vi "Initialise Singleton.vi"(8 "error in (no error)":errorcluster, 11 "Class in":refnum<class>) -> (0 "error out":errorcluster)   [LabVIEW 2020, in "Singleton.lvlib"]
uses:
  Singleton.lvlib
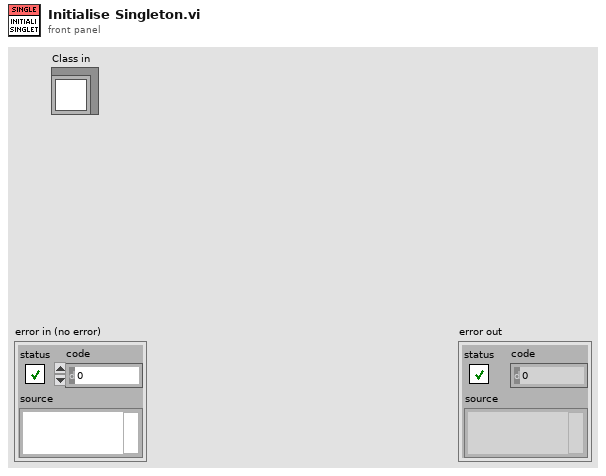
[diagram p1: front panel]
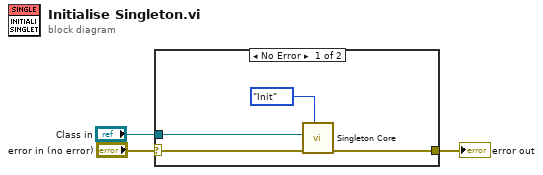
[diagram p0: block diagram]
diagram:
  n1 = case shown="No Error" "error in (no error)" {
    selector: "error in (no error)" -> [w7 w8]
    tunnel: [w6 w8] -> w2
    tunnel: "Class in" -> [w4 _]
    frame No Error {
      n2 = call "Singleton Core.vi"("Action"=enum16{"Init", "Write Object", "Read Object"}."Init", "error in (no error)"=w7, "Class in"=w4) -> ("error out"=w6:errorcluster)  [unwired: 7 in, 1 out]
    }
    frame Error {
    }
  }
  "error out" <- w2
